vi "Initialize.vi"(8 "error in":errorcluster, 11 "Plugin in":refnum<class "Historical Table.lvclass">) -> (0 "error out":errorcluster, 3 "Plugin out":refnum<class "Historical Table.lvclass">)   [LabVIEW 2024, in "Historical Table.lvlib" / "Historical Table.lvclass"]
uses:
  Historical Table.lvclass
  C:/Program Files/National Instruments/LabVIEW 2024/vi.lib/FlexLogger/SDK/PluginSDK.lvlibp/PEFClasses/SDK/Plugin/Plugin.lvclass
  <vilib>/FlexLogger/SDK/PluginSDK.lvlibp/PEFClasses/SDK/System Interface/Resampling Mode.ctl
  <vilib>/FlexLogger/SDK/PluginSDK.lvlibp/PEFClasses/SDK/Processing Element/Timing Parameters.ctl
  <vilib>/FlexLogger/SDK/PluginSDK.lvlibp/PEFClasses/SDK/Processing Element/Timing Method.ctl
  Historical Table.lvclass/Historical Table.ctl
  Global Strings.vi
  <vilib>/FlexLogger/SDK/PluginSDK.lvlibp/PEFClasses/SDK/Plugin/ParameterAccess/Write N Channel.vi
  <vilib>/FlexLogger/SDK/PluginSDK.lvlibp/PEFClasses/SDK/Plugin/ParameterAccess/Write I32.vi
  <vilib>/FlexLogger/SDK/PluginSDK.lvlibp/PEFClasses/SDK/Plugin/ParameterAccess/Write Command.vi
  Historical Table UI.vi
  <vilib>/FlexLogger/SDK/PluginSDK.lvlibp/PEFClasses/SDK/Plugin/Plugin.lvclass
  <vilib>/FlexLogger/SDK/PluginSDK.lvlibp/PEFClasses/SDK/System Interface/System Interface.lvclass
  <vilib>/FlexLogger/SDK/PluginSDK.lvlibp/PEFClasses/SDK/Processing Element/Processing Element.lvclass
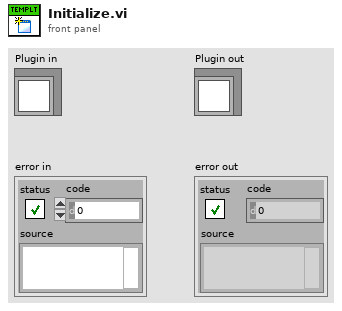
[diagram p1: front panel]
types:
  T1 = typedef "PluginSDK.lvlibp/Processing Element.lvclass/Timing Parameters.ctl" = cluster{"Timing Method":T2, "Timing Period (ms)":i32}
  T2 = typedef "PluginSDK.lvlibp/Processing Element.lvclass/Timing Method.ctl" = enum16{"Periodic", "Immediate", "On Data Ready", "Triggered"}
  T3 = typedef "PluginSDK.lvlibp/System Interface.lvclass/Resampling Mode.ctl" = enum16{"No Resampling", "Custom Rate", "Maximum Rate", "Minimum Rate"}
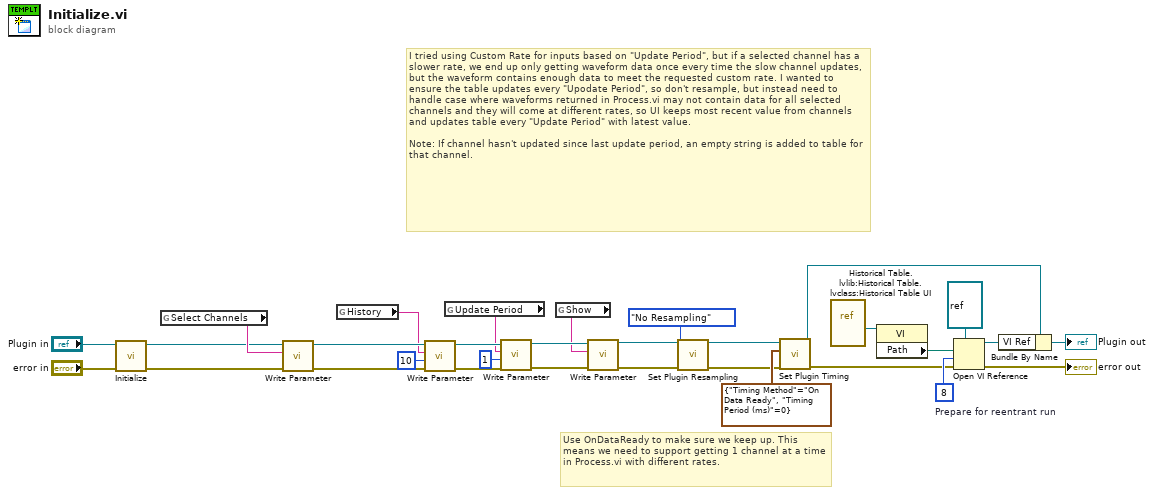
[diagram p0: block diagram]
diagram:
  w7 = 8  # Prepare for reentrant run
  # "Use OnDataReady to make sure we keep up. This means we need to support getting 1 channel at a time in Process.vi with different rates."
  # "I tried using Custom Rate for inputs based on \"Update Period\", but if a selected channel has a slower rate, we end up only getting waveform data once every time the slow channel updates, but the waveform contains enough data to meet the requested custom rate. I wanted to ensure the table updates every \"Upodate Period\", so don't resample, but instead need to handle case where waveforms returned in Process.vi may not contain data for all selected channels and they will come at different rates, so UI keeps most recent value from channels and updates table every \"Update Period\" with latest value.\n\nNote: If channel hasn't updated since last update period, an empty string is added to table for that channel."
  n1 = call-parent "Initialize.vi"("error in (no error)"="error in", "Plugin in"="Plugin in") -> ("error out"=w16:errorcluster, "Plugin out"=w17:refnum<class "Historical Table.lvclass">)  [unwired: 8 in]
  n2 = global read "Global Strings.vi" "Select Channels"() -> (w23:string)
  n3 = call-poly <vilib>:"Write Parameter.vi"("error in (no error)"=w16, "Name (Unique Channel Identifier)"=w23, "Plugin in"=w17) -> ("error out"=w28:errorcluster, "Plugin out"=w29:refnum<class "Historical Table.lvclass">)  [unwired: 7 in]
  n4 = global read "Global Strings.vi" "History"() -> (w22:string)
  n5 = call-poly <vilib>:"Write Parameter.vi"("error in (no error)"=w28, "Value"=10, "Name"=w22, "Plugin in"=w29) -> ("error out"=w25:errorcluster, "Plugin out"=w26:refnum<class "Historical Table.lvclass">)  [unwired: 6 in]
  n6 = global read "Global Strings.vi" "Update Period"() -> (w21:string)
  n7 = call-poly <vilib>:"Write Parameter.vi"("error in (no error)"=w25, "Value"=1, "Name"=w21, "Plugin in"=w26) -> ("error out"=w18:errorcluster, "Plugin out"=w20:refnum<class "Historical Table.lvclass">)  [unwired: 6 in]
  n8 = global read "Global Strings.vi" "Show"() -> (w19:string)
  n9 = call-poly <vilib>:"Write Parameter.vi"("error in (no error)"=w18, "Name"=w19, "Plugin in"=w20) -> ("error out"=w10:errorcluster, "Plugin out"=w11:refnum<class "Historical Table.lvclass">)  [unwired: 7 in]
  n10 = call <vilib>:"Set Plugin Resampling.vi"("Plugin in"=w11, "Resampling Mode"=Resampling_Mode."No Resampling", "error in (no error)"=w10) -> ("Plugin out"=w13:refnum<class "Historical Table.lvclass">, "error out"=w12:errorcluster)  [unwired: 11 in]
  n11 = call <vilib>:"Set Plugin Timing.vi"("error in (no error)"=w12, "Timing Parameters"=T1 {"Timing Method"=enum."On Data Ready", "Timing Period (ms)"=0}, "Plugin in"=w13) -> ("error out"=w5:errorcluster, "Plugin out"=w4:refnum<class "Historical Table.lvclass">)  [unwired: 7 in]
  n12 = vi-ref "Historical Table.lvlib:Historical Table.lvclass:Historical Table UI.vi"() -> (w9:refnum<vi>)
  n13 = property class="VI"(reference=w9) -> ("Path"=w8:path)  [unwired: 1 in, 2 out]
  n14 = Open VI Reference(type specifier VI Refnum (for type only)=refnum<vi> refnum, vi path=w8, options=w7, error in (no error)=w5) -> (vi reference=w3:refnum<vi>, error out=→"error out":errorcluster)  [unwired: 2 in]
  n15 = Bundle By Name(cluster=w4, "VI Ref"=w3) -> (→"Plugin out":refnum<class "Historical Table.lvclass">)
